vi "Lectura archivos RPS para análisis.vi"(8 "error in (no error)":errorcluster, 11 "Ruta archivo a analizar":path) -> (0 "error out":errorcluster, 1 "Temperaturas":T1, 2 "Cadena de datos":string, 3 "Tamaño Archivo":i64)   [LabVIEW 2012]
doc: "Este Vi lee archivos de datos del sistema de resonancia de plasmones, extrae la cadena con los datos en ascii y obtiene la información referente a la temperatura inicial y final"
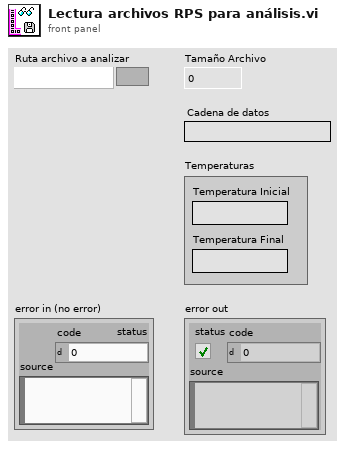
[diagram p1: front panel]
types:
  T1 = cluster{"Temperatura Inicial":string, "Temperatura Final":string}
  T2 = enum16{"open", "replace", "create", "open or create", "replace or create", "replace or create with confirmation"}
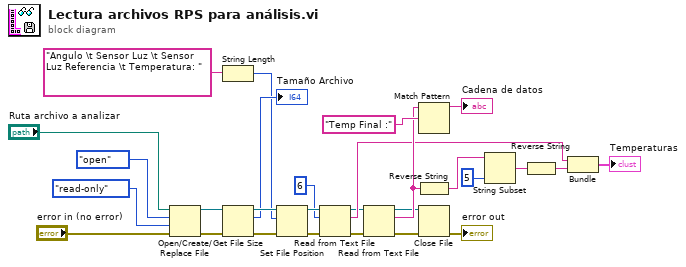
[diagram p0: block diagram]
diagram:
  n1 = Open/Create/Replace File(file path (use dialog)="Ruta archivo a analizar", error in="error in (no error)", operation (0:open)=T2."open", access (0:read/write)=enum16{"read/write", "read-only", "write-only"}."read-only") -> (refnum out=w11:refnum<file>, error out=w10:errorcluster)  [unwired: 2 in, 1 out]
  n2 = String Length(string="Angulo \t Sensor Luz \t Sensor Luz Referencia \t Temperatura: ") -> (length=w8:i32)
  n3 = Get File Size(file=w11, error in=w10) -> (refnum out=w13:refnum<file>, size (in bytes)=→"Tamaño Archivo":i64, 0:w14:errorcluster)
  n4 = Set File Position(offset (in bytes) (0)=w8, refnum=w13, error in=w14) -> (refnum out=w7:refnum<file>, error out=w5:errorcluster)  [unwired: 1 in]
  n5 = Read from Text File(file (use dialog)=w7, count=6, error in=w5) -> (refnum out=w4:refnum<file>, text=w23:string, error out=w3:errorcluster)  [unwired: 1 in, 1 out]
  n6 = Read from Text File(file (use dialog)=w4, error in=w3) -> (refnum out=w16:refnum<file>, text=w26:string, error out=w15:errorcluster)  [unwired: 2 in, 1 out]
  n7 = Match Pattern(string=w26, regular expression="Temp Final :") -> (before substring=→"Cadena de datos":string)  [unwired: 1 in, 3 out]
  n8 = Reverse String(1:w26) -> (0:w19:string)
  n9 = Close File(refnum=w16, error in=w15) -> (error out=→"error out":errorcluster)  [unwired: 1 out]
  n10 = String Subset(string=w19, length (rest)=5 ("length (rest)")) -> (substring=w21:string)  [unwired: 1 in]
  n11 = Reverse String(1:w21) -> (0:w25:string)
  n12 = Bundle(w23, w25) -> (→"Temperaturas":cluster{string, string})  [unwired: 1 in]
